vi "Generate Display Manager DVR.vi"(8 "Error In":errorcluster, 11 "Display Manager In":refnum<class "Display Manager.lvclass">) -> (0 "Error Out":errorcluster, 3 "Display Manager Out":refnum<class "Display Manager.lvclass">)   [LabVIEW 2021, in "Display Manager.lvclass"]
uses:
  Display Manager.lvclass
  Controls/Data.ctl
  Display Utilities/Public/Controls/2D Dimensions.ctl
  Display Manager.lvclass/Display Manager.ctl
  Display Utilities/Display Utilities.lvlib
  Display Element/Display Element.lvclass
  Animation/Animation.lvclass
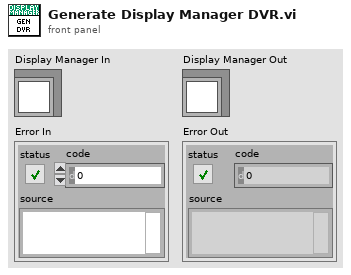
[diagram p1: front panel]
types:
  T1 = typedef "Display Manager.lvclass/Data.ctl" = cluster{"Size":T2, "Display Elements":refnum<class "Display Element.lvclass">[], "Frame":u32[][], "Animations":refnum<class "Animation.lvclass">[]}
  T2 = typedef "Display Utilities.lvlib/2D Dimensions.ctl" = cluster{"Width":i32, "Height":i32}
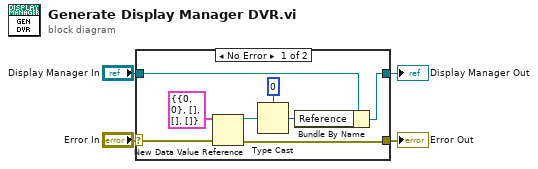
[diagram p0: block diagram]
diagram:
  n1 = case shown="No Error" "Error In" {
    selector: "Error In" -> [w11 w14]
    tunnel: "Display Manager In" -> [w8 w13]
    tunnel: [w5 w14] -> w2
    tunnel: [w6 w13] -> w1
    frame No Error {
      n2 = New Data Value Reference(data value=T1 {"Size"={"Width"=0, "Height"=0}, "Display Elements"=[], "Frame"=[], "Animations"=[]} ("Data"), error in=w11) -> (data value reference=w9:refnum<data-value>, error out=w5:errorcluster)
      n3 = Type Cast(type=u64 0, x=w9) -> (*(type *) &x=w7:u64)
      n4 = Bundle By Name(cluster=w8, "Reference"=w7) -> (w6:refnum<class "Display Manager.lvclass">)
    }
    frame Error {
    }
  }
  "Display Manager Out" <- w1
  "Error Out" <- w2
